vi "SetPorts.vi"() -> (0 "Ports":T1={"Flow Controllers"="COM1", "Oven Fan"="COM9", "Oven Watlows"="COM4", "Field Power Supply"="COM3"})   [LabVIEW 2009]
uses:
  <vilib>/Instr/_visa.llb/VISA Configure Serial Port (Instr).vi
panel:
  in  "Ports":T1={"Flow Controllers"="COM1", "Oven Fan"="COM9", "Oven Watlows"="COM4", "Field Power Supply"="COM3"}
  in  "Field Power Supply":refnum<visa-resource-name>="COM3"
  in  "Oven Watlows":refnum<visa-resource-name>="COM4"
  in  "Oven Fan":refnum<visa-resource-name>="COM9"
  in  "Flow Controllers":refnum<visa-resource-name>="COM1"
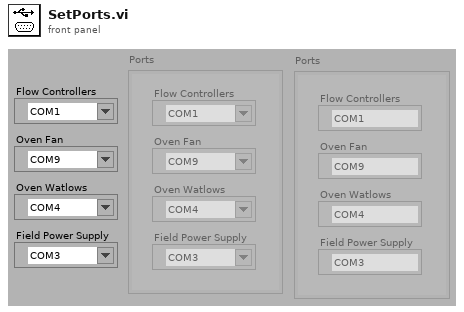
[diagram p1: front panel]
types:
  T1 = cluster{"Flow Controllers":refnum<visa-resource-name>, "Oven Fan":refnum<visa-resource-name>, "Oven Watlows":refnum<visa-resource-name>, "Field Power Supply":refnum<visa-resource-name>}
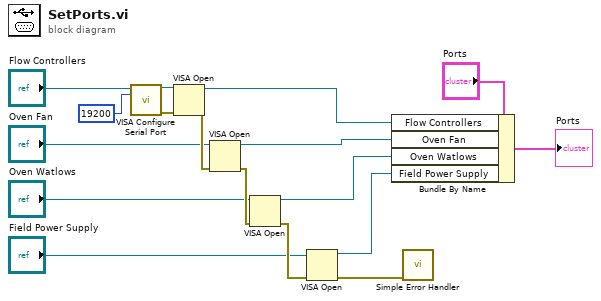
[diagram p0: block diagram]
diagram:
  n1 = call-poly "VISA Configure Serial Port"("VISA resource name"="Flow Controllers", "baud rate (9600)"=19200) -> ("VISA resource name out"=w14:refnum<visa-resource-name>, "error out"=w12:errorcluster)  [unwired: 4 in, 8 out]
  n2 = VISA Open(error in (no error)=w12, VISA resource name=w14) -> (VISA resource name=w13:refnum<visa-resource-name>, error out=w11:errorcluster)  [unwired: 3 in]
  n3 = VISA Open(error in (no error)=w11, VISA resource name="Oven Fan") -> (VISA resource name=w2:refnum<visa-resource-name>, error out=w10:errorcluster)  [unwired: 3 in]
  n4 = VISA Open(error in (no error)=w10, VISA resource name="Oven Watlows") -> (VISA resource name=w4:refnum<visa-resource-name>, error out=w9:errorcluster)  [unwired: 3 in]
  n5 = VISA Open(error in (no error)=w9, VISA resource name="Field Power Supply") -> (VISA resource name=w6:refnum<visa-resource-name>, error out=w8:errorcluster)  [unwired: 3 in]
  n6 = Bundle By Name(cluster="Ports", "Flow Controllers"=w13, "Oven Fan"=w2, "Oven Watlows"=w4, "Field Power Supply"=w6) -> (→"Ports":T1)
  n7 = call <vilib>:"Simple Error Handler.vi"("error in (no error)"=w8) -> ()  [unwired: 4 in, 5 out]
